vi "R_Run.vi"(8 "错误输入（无错误）":errorcluster, 11 "队列输入":refnum<queue>) -> ()   [LabVIEW 2018]
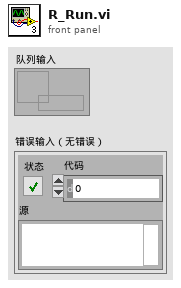
[diagram p1: front panel]
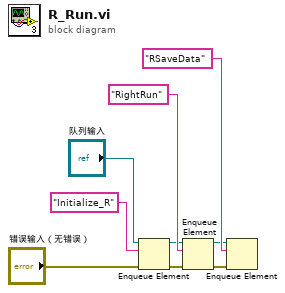
[diagram p0: block diagram]
diagram:
  n1 = Enqueue Element(queue="队列输入", element="Initialize_R", error in (no error)="错误输入（无错误）") -> (queue out=w1:refnum<queue>, error out=w2:errorcluster)  [unwired: 1 in, 1 out]
  n2 = Enqueue Element(queue=w1, element="RightRun", error in (no error)=w2) -> (queue out=w4:refnum<queue>, error out=w5:errorcluster)  [unwired: 1 in, 1 out]
  n3 = Enqueue Element(queue=w4, element="RSaveData", error in (no error)=w5) -> ()  [unwired: 1 in, 3 out]
